vi "main OP400.vi"() -> ()   [LabVIEW 2020]
uses:
  SubVI/OP400ZP_state.ctl
  <userlib>/Alex.vi/FGV.ctl
  <vilib>/QMT/GDataBase for MySQL(tm)/MySQL/public/controls/DateType.ctl
  OP500/VG/VG_progressBar.vi
  OP600/SubVI/CheminDeBase.vi
  <vilib>/Utility/error.llb/Error Cluster From Error Code.vi
  VG/PN.vi
  VG/ZENTYPE.vi
  VG/IS30%.vi
  OP300/EN PRODUCTION/OP300-CONTI-AUTO/VG/R.vi
  VG/VG_BT3562.vi
  SubVI/OP400ZP_OCVmin.vi
  SubVI/OP400ZP_OCVmax.vi
  VG/VG_MX5060.vi
  <vilib>/Instr/_visa.llb/VISA Configure Serial Port (Instr).vi
  VG/VG_ARDUINO.vi
  <vilib>/QMT/GDataBase for MySQL(tm)/MySQL/MySQLConnector.lvclass
panel:
  out "error out":errorcluster
  out "INSERT INTO":string
  out "Revision":i32=288
  out "BDD 2":T1
  in  "arrêt":bool
  out "BT3562A":refnum<visa-resource-name>
  out "MX5060":refnum<visa-resource-name>
  in  "VISA OUT":T2
  out "VISA OUT":T2
  out "Compt":i32
  in  "DERNIER2":bool
  out "30% ?":bool
  out "SN":string
  out "Zentype":string
  out "BDD":T3
  out "Numérique":i32
  out "progression":dbl(slide) scale=0.0..1000.0
  out "PN":string
  out "errout 2":errorcluster={"status"=TRUE, "code"=0, "source"="PCAN_CHANNEL ILLEGAL"} caption="errout"
  out "errout":errorcluster caption="sortie d'erreur"
  out "STOP":bool
  out "TOP":string
  out "DRAW":picture
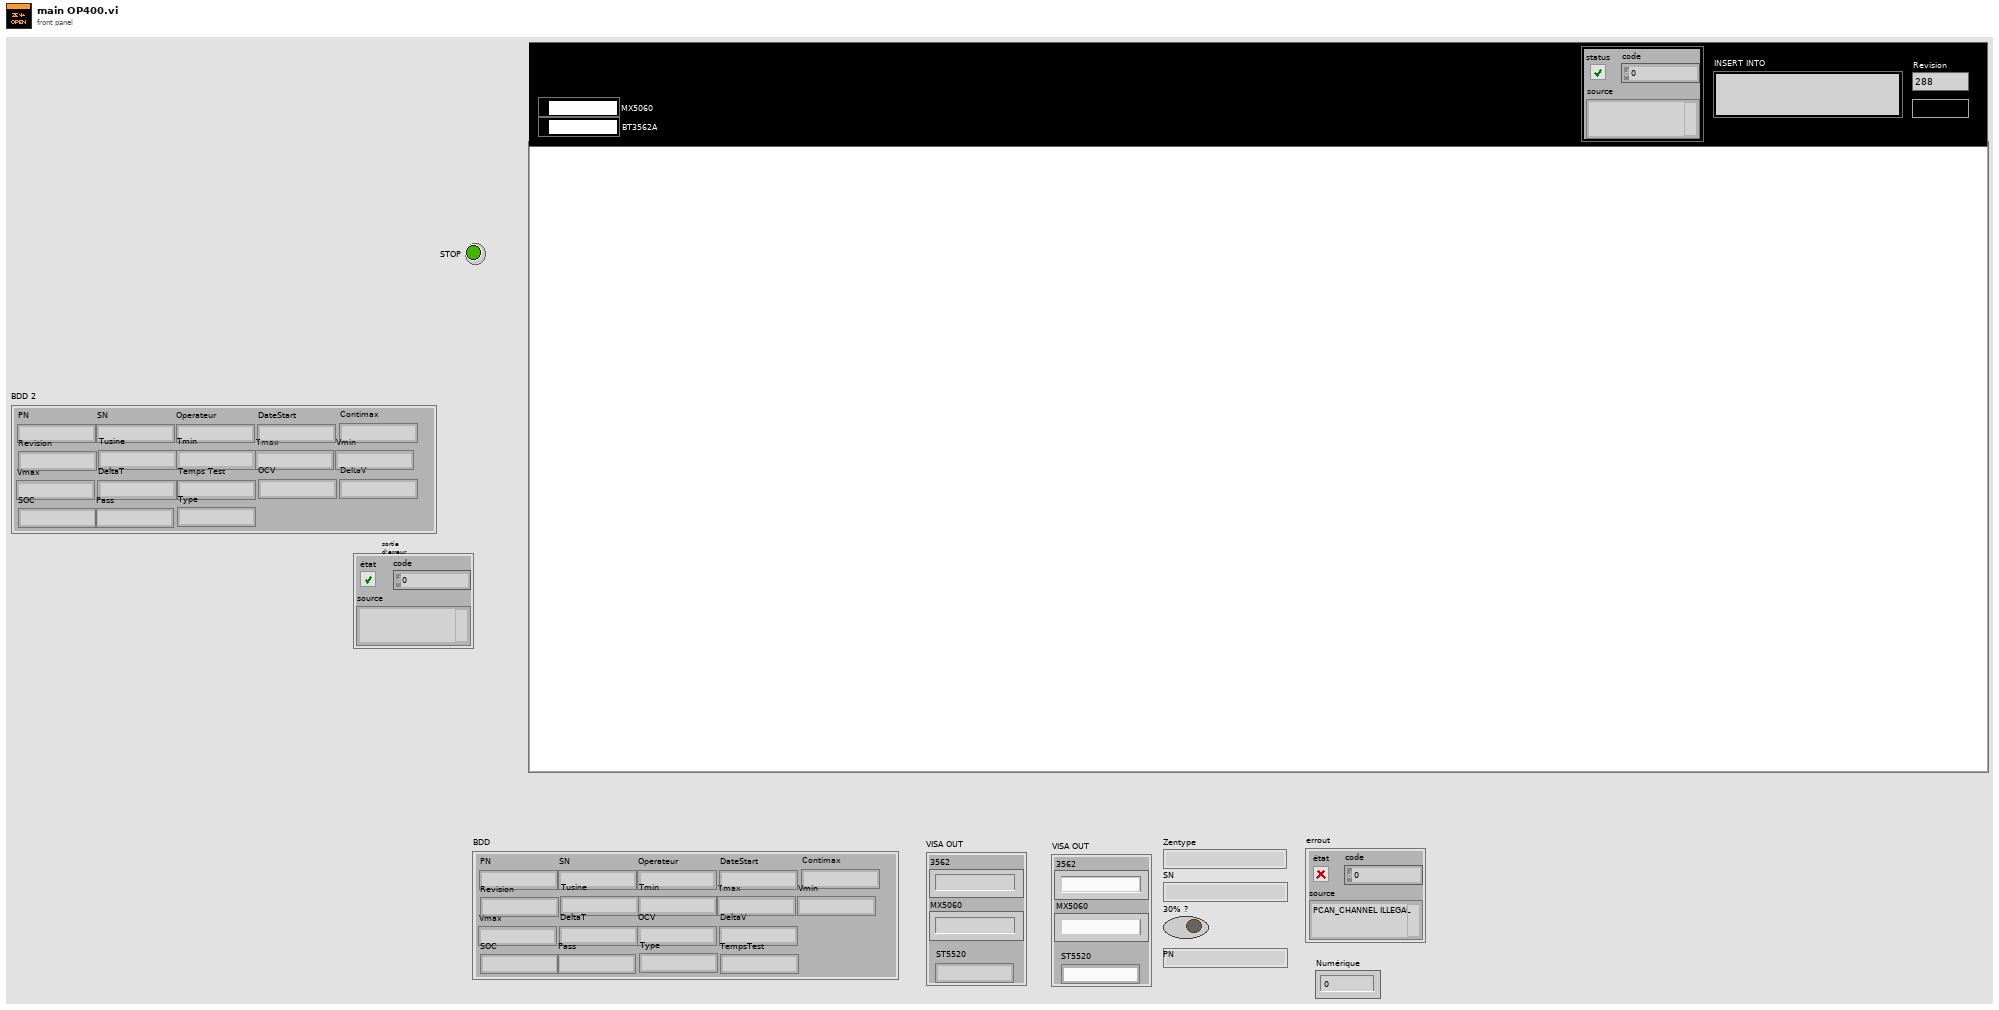
[diagram p1: front panel]
types:
  T1 = cluster{"Operateur":string, "DateStart":string, "Contimax":string, "PN":string, "Revision":string, "Tusine":string, "Tmin":string, "Tmax":string, "Vmin":string, "Vmax":string, "DeltaT":string, "Temps Test":string, "OCV":string, "SN":string, "DeltaV":string, "SOC":string, "Pass":string, "Type":string}
  T2 = cluster{"3562":string, "MX5060":string, "ST5520":string}
  T3 = cluster{"PN":string, "SN":string, "Operateur":string, "DateStart":string, "Contimax":string, "Revision":string, "Tusine":string, "Tmin":string, "Tmax":string, "Vmin":string, "Vmax":string, "DeltaT":string, "OCV":string, "DeltaV":string, "SOC":string, "Pass":string, "Type":string, "TempsTest":string}
  T4 = cluster{"PN":string, "Opérateur":string, "Sealing":string, "Conti":string, "OCV":string, "1_TCellmin":string, "1_TCellmax":string, "1_VCellmin":string, "1_VCellmax":string, "1_Nbmodule":string, "Résultat final":string, "Résultat final 2":string, "1_Nbmodule 2":string, "1_VCellmax 2":string, "Résultat final 3":string, "1_Nbmodule 3":string, "Résultat final 4":string, "1_Nbmodule 4":string, "1_VCellmax 3":string, "Résultat final 5":string}
  T5 = typedef "OP400ZP_state.ctl" = enum16{"Null", "Demarrage", "Init", "Scan", "Montage", "Conti", "Iso", "Vpack", "DataDyn", "Demontage", "Crash", "Next", "Sealing", "Comext"}
  T6 = typedef "FGV.ctl" = enum16{"GET", "SET", "RAZ"}
  T7 = typedef "MySQLVIEW.lvlib/MySQLConnector.lvclass/DateType.ctl" = enum16{"DATETIME", "DATE", "TIMESTAMP", "TIME", "YEAR (2 digits)", "YEAR (4 digits)"}
  T8 = enum32{"BT3561A", "BT3562A", "BT3563A", "BT3562", "BT3563", "BT3564", "3561"}
  T9 = cluster{"1_TCellmin":string, "1_TCellmax":string, "1_VCellmin":string, "1_VCellmax":string, "1_Nbmodule":string, "1_TUsine":string, "1_DeltaT":string, "1_DeltaV":string}
  T10 = typedef "imagedata.ctl" = cluster{"image type":i32, "image depth":i32, "image":u8[], "mask":u8[], "colors":u32[], "Rectangle":cluster{"left":i16, "top":i16, "right":i16, "bottom":i16}}
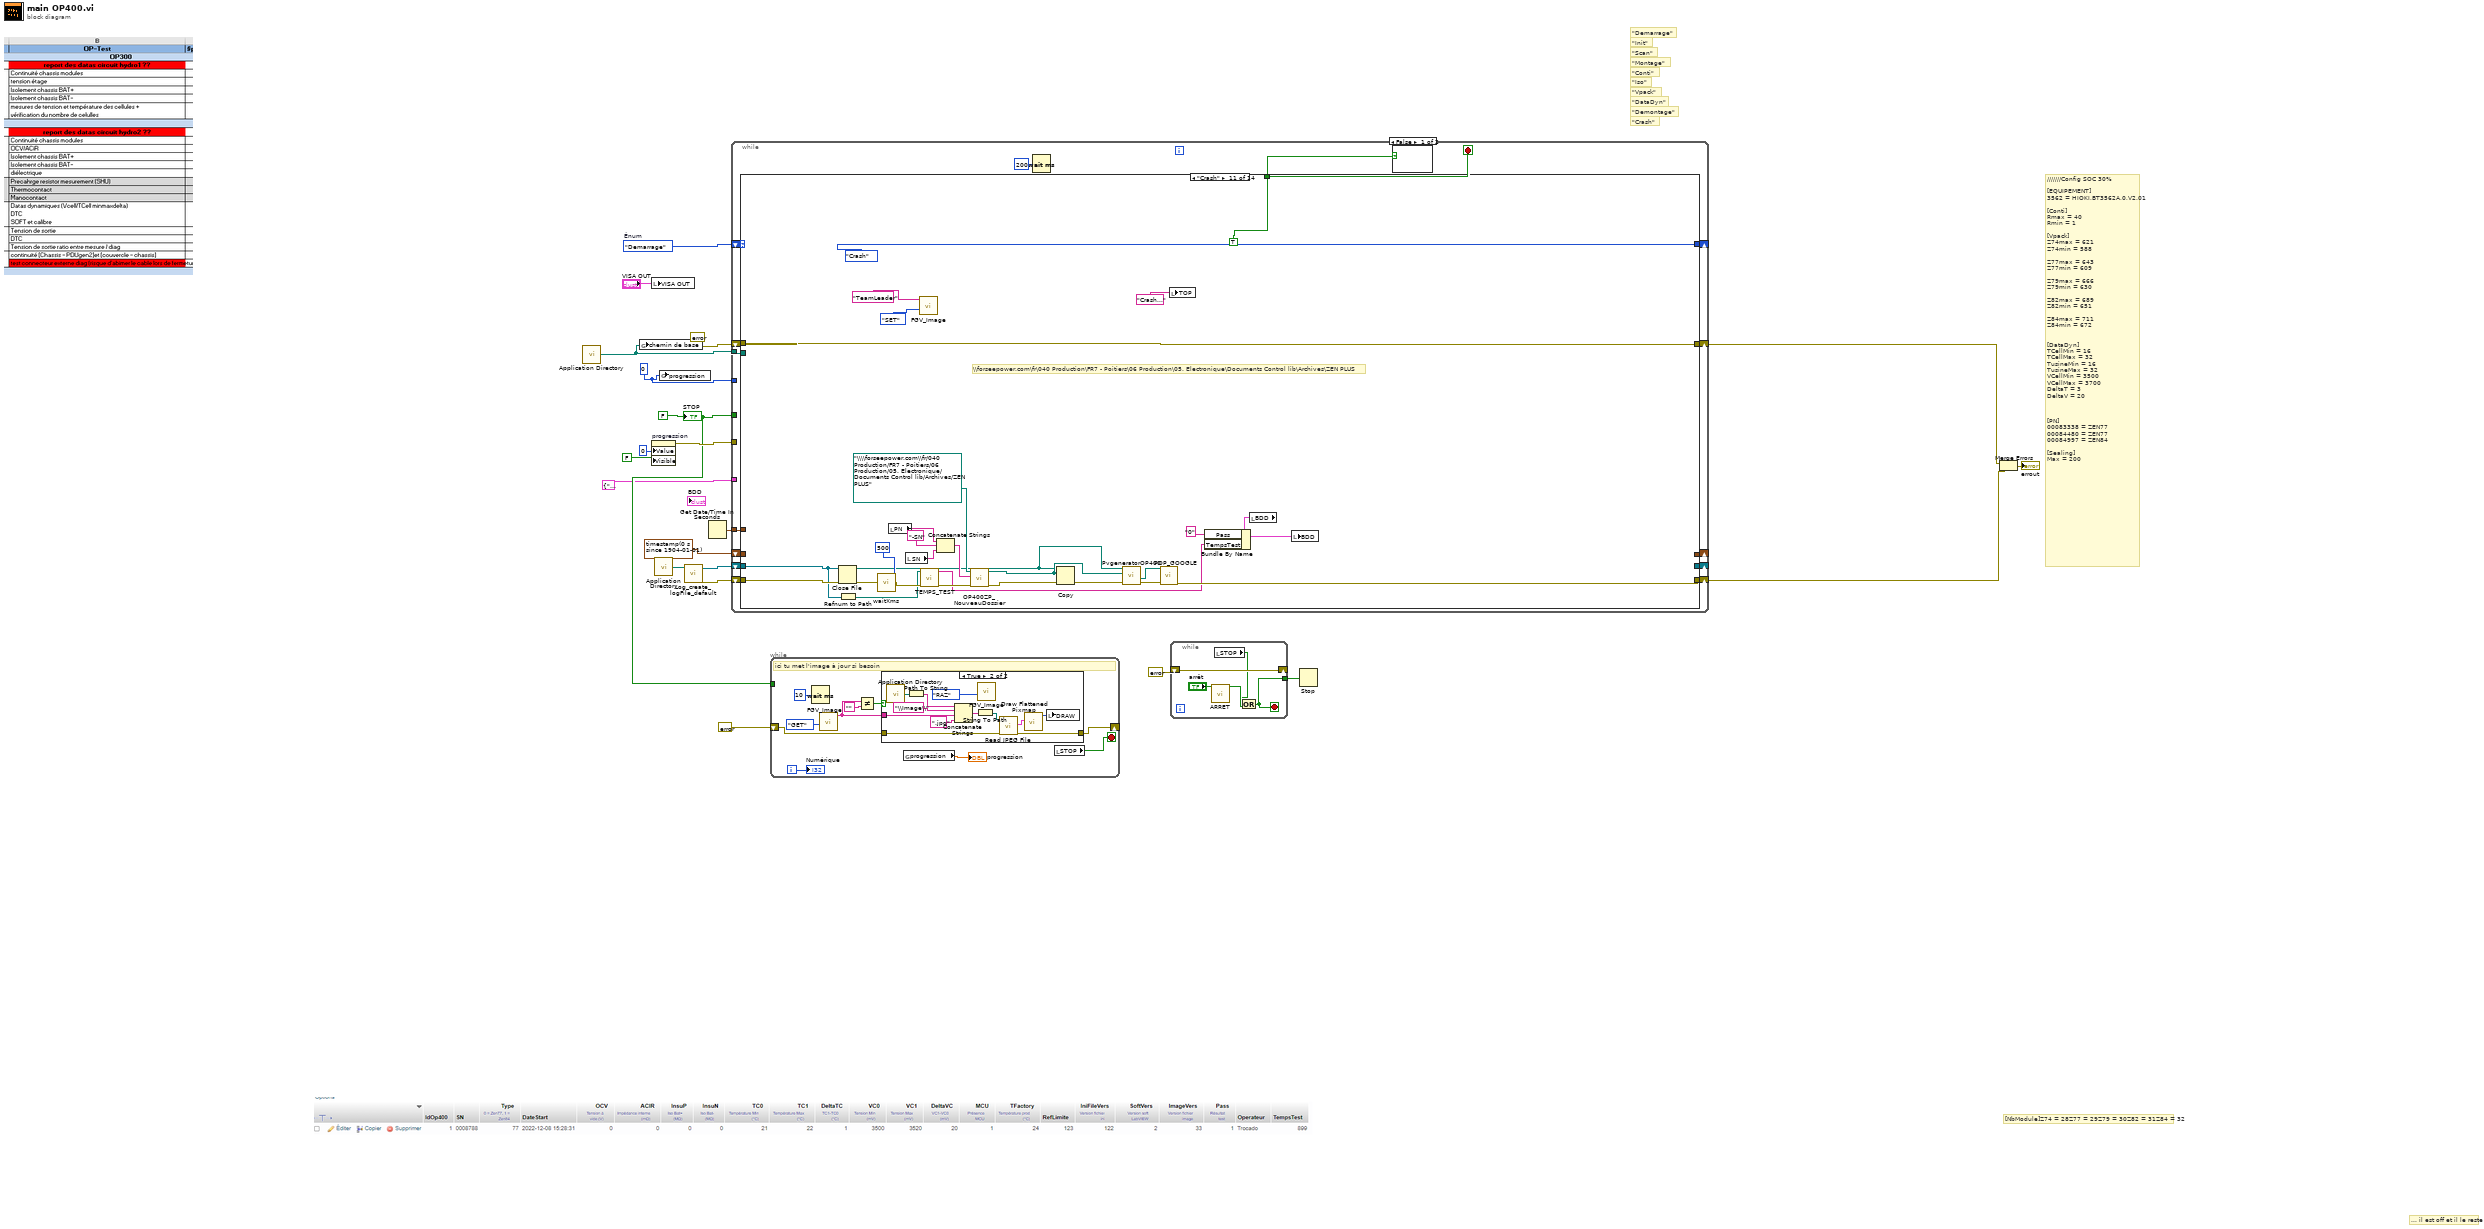
[diagram p0: block diagram]
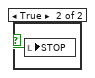
[diagram p3: hidden frame]
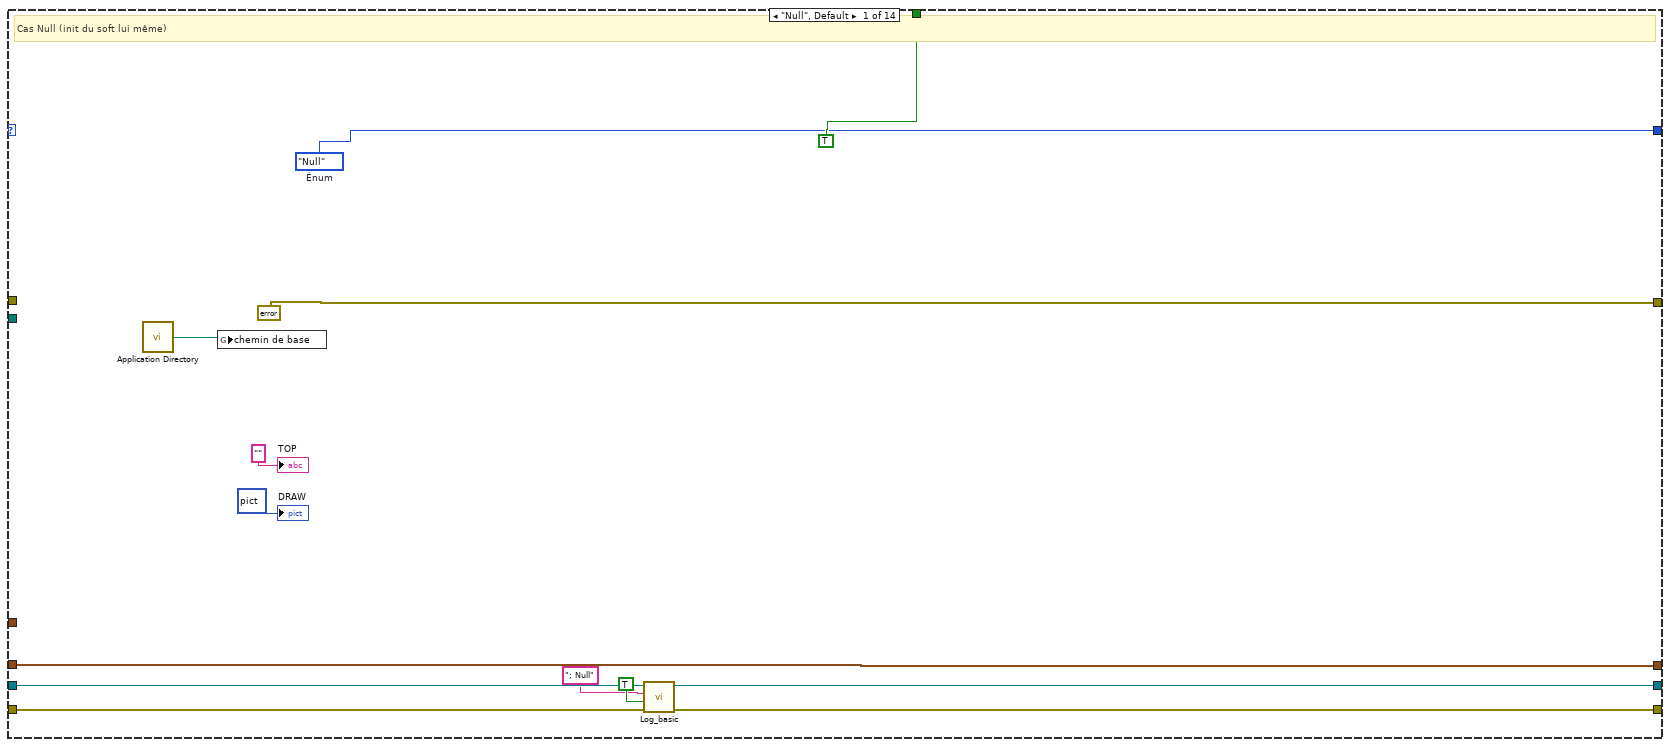
[diagram p4: hidden frame]
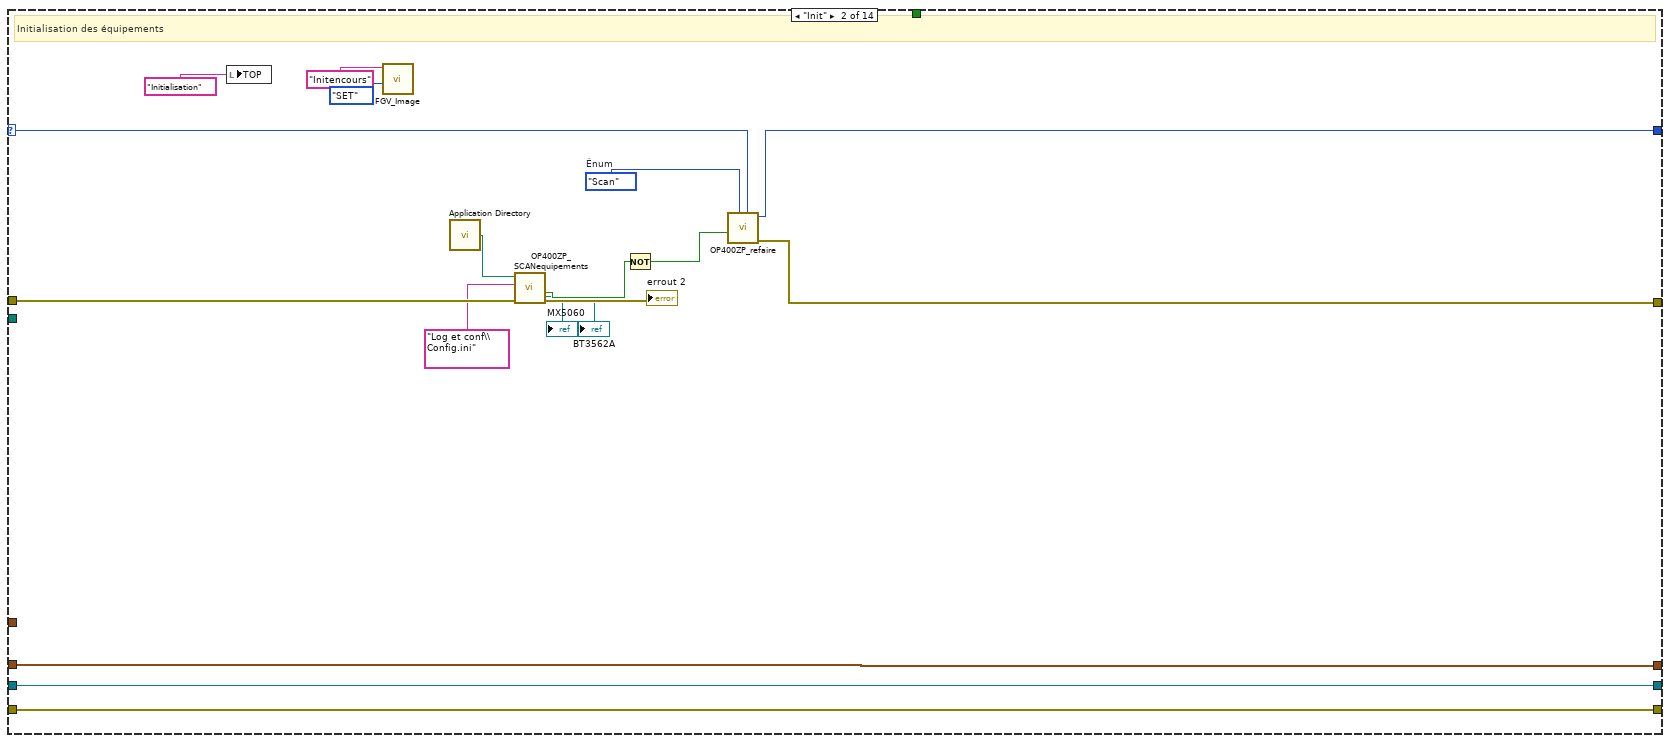
[diagram p5: hidden frame]
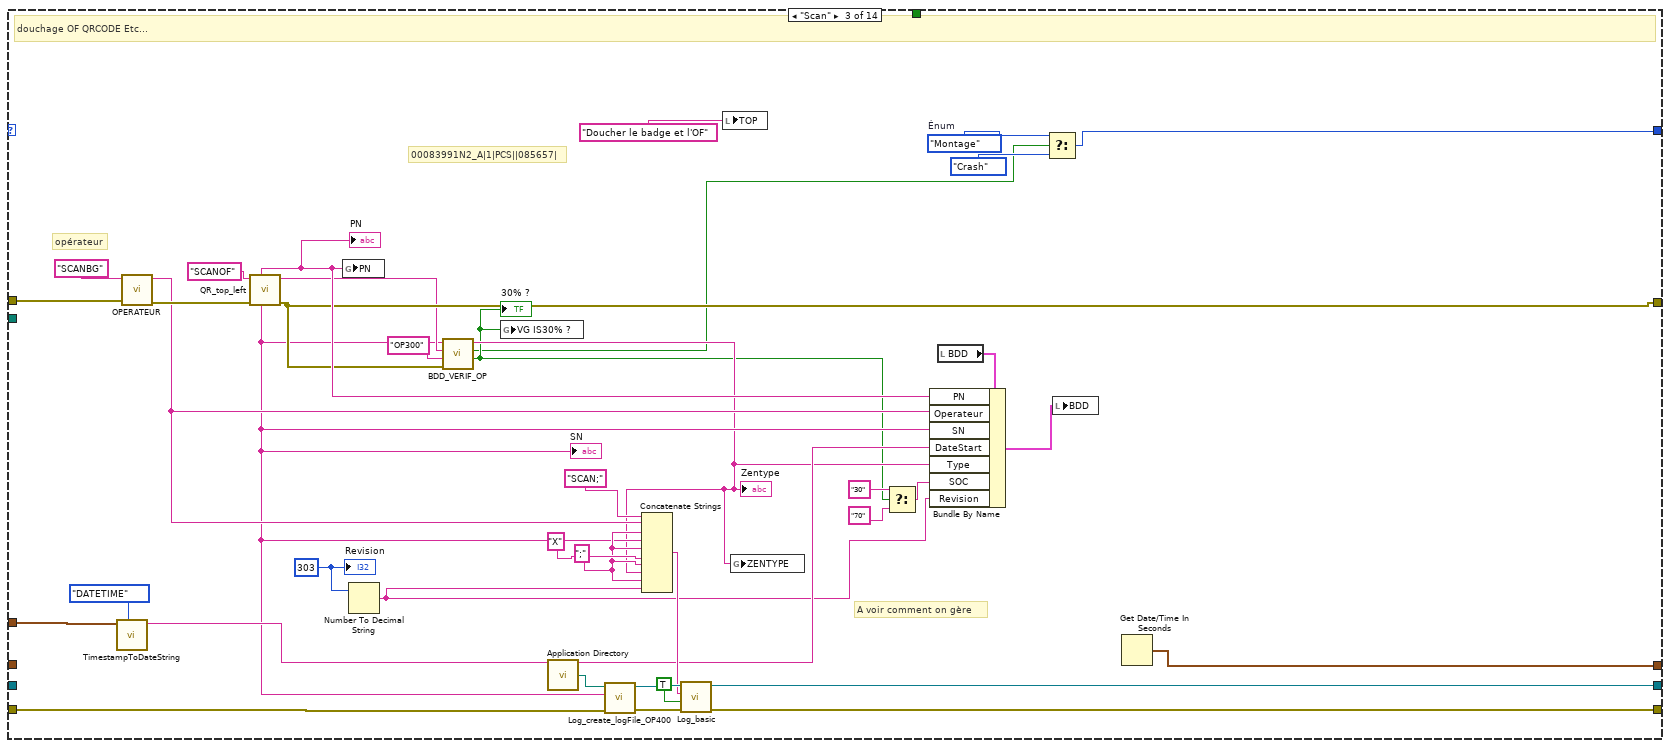
[diagram p6: hidden frame]
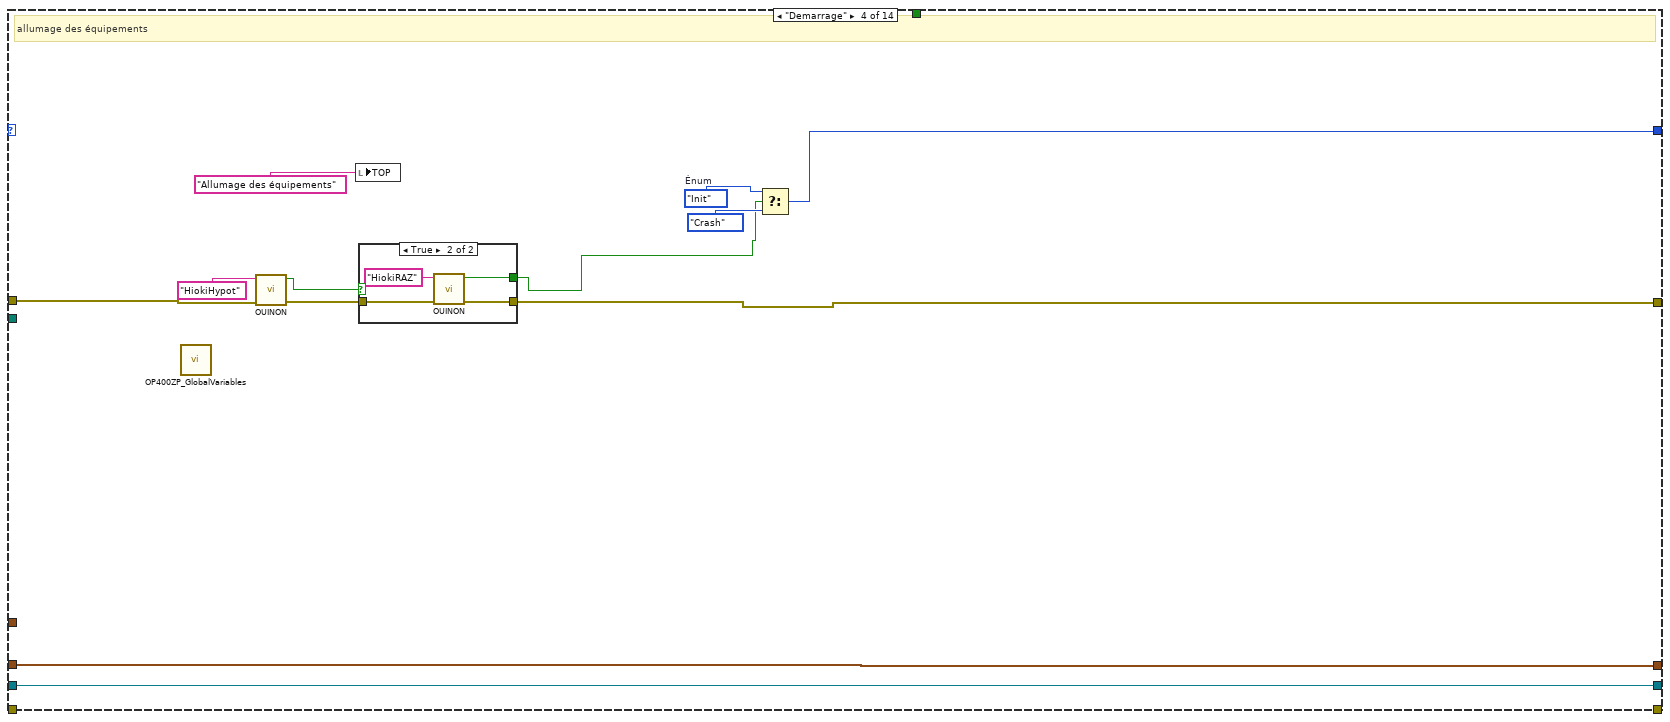
[diagram p7: hidden frame]
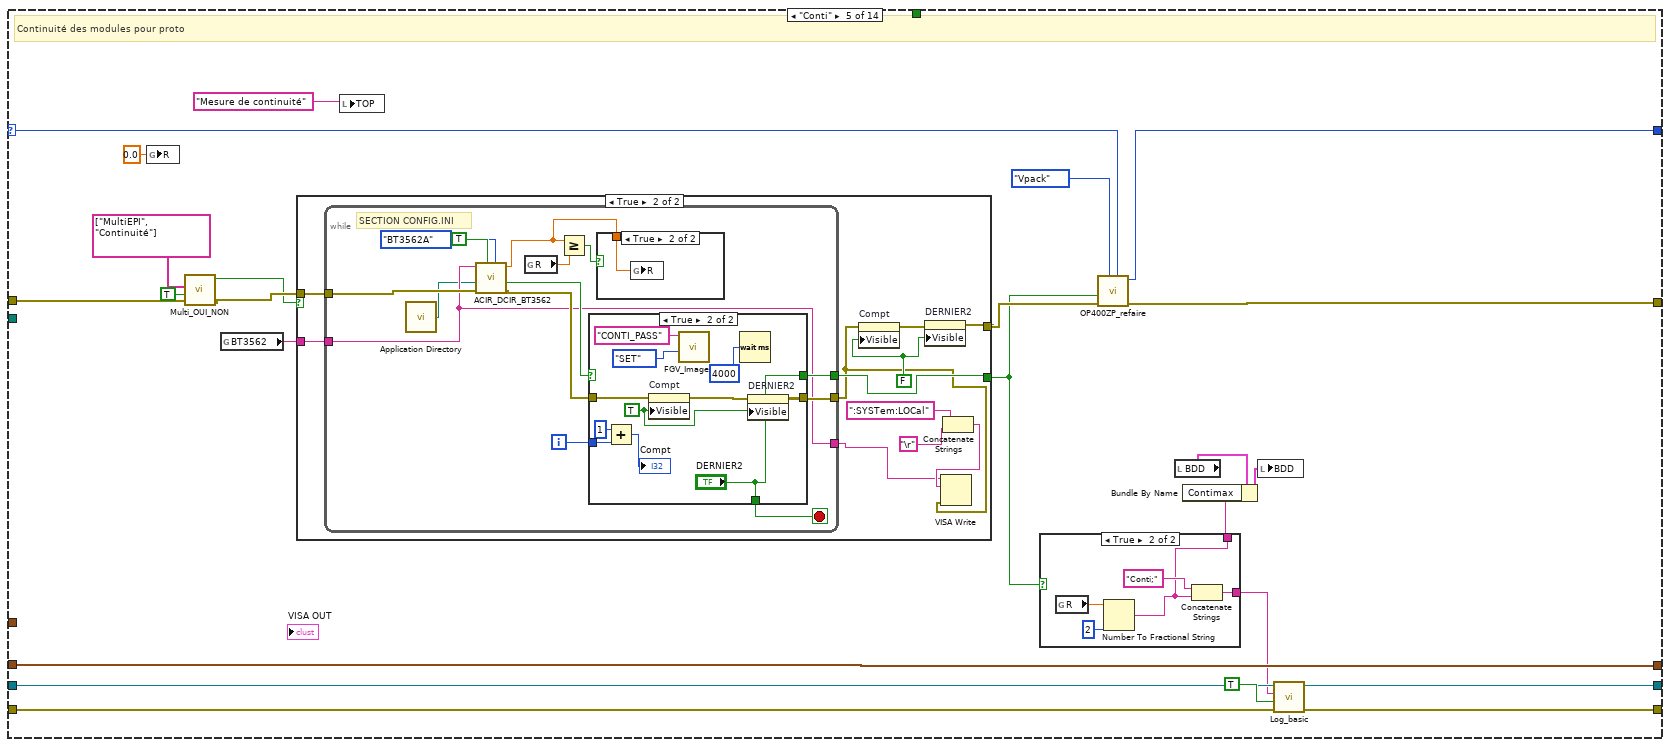
[diagram p9: hidden frame]
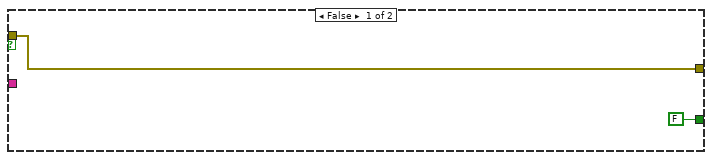
[diagram p10: hidden frame]
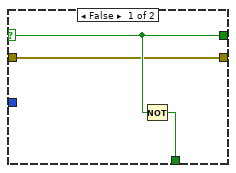
[diagram p11: hidden frame]
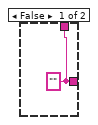
[diagram p13: hidden frame]
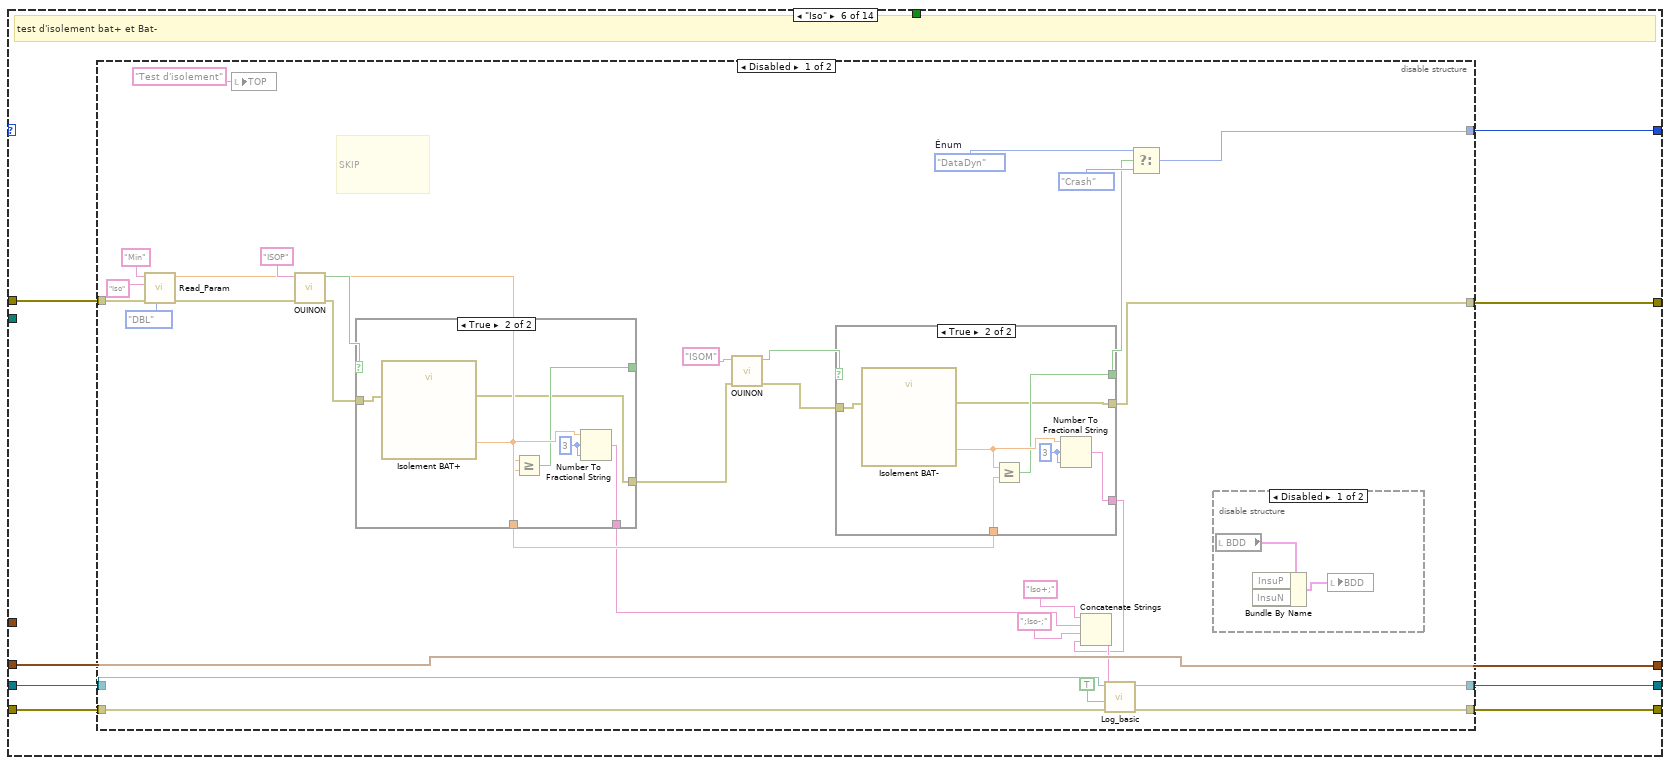
[diagram p14: hidden frame]
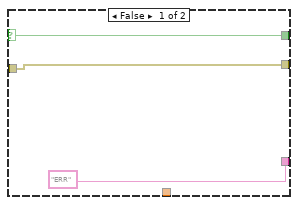
[diagram p16: hidden frame]
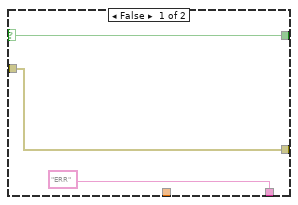
[diagram p17: hidden frame]
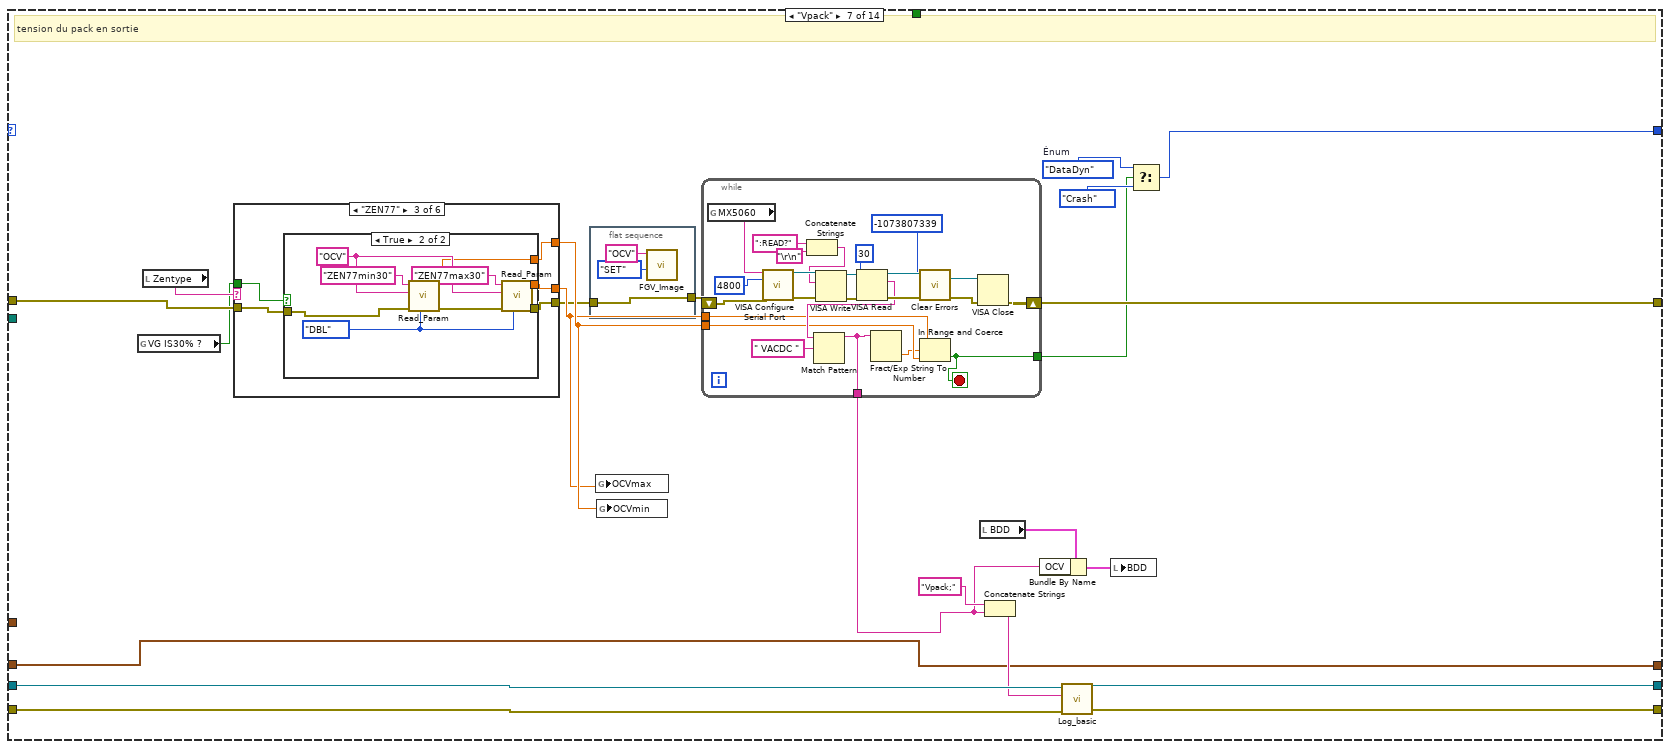
[diagram p19: hidden frame]
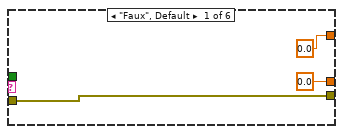
[diagram p20: hidden frame]
diagram:
  w1 = u8 0 ("progression")
  w12 = OP400ZP_state."Demarrage"  # Énum
  w7 = FALSE ("STOP")
  # "[NbModule]Z74 = 28Z77 = 29Z79 = 30Z82 = 31Z84 = 32"
  # "///////Config SOC 30%\n\n[EQUIPEMENT]\n3562 = HIOKI,BT3562A,0,V2.01\n\n[Conti]\nRmax = 40\nRmin = 1\n\n[Vpack]\nZ74max = 621\nZ74min = 588\n\nZ77max = 643\nZ77min = 609\n\nZ79max = 666\nZ79min = 630\n\nZ82max = 689\nZ82min = 651\n\nZ84max = 711\nZ84min = 672\n\n\n[DataDyn]\nTCellMin = 16\nTCellMax = 32\nTusineMin = 16\nTusineMax = 32\nVCellMin = 3500\nVCellMax = 3700\nDeltaT = 3\nDeltaV = 20\n\n\n\n[PN]\n00083338 = ZEN77\n00084480 = ZEN77\n00084997 = ZEN84\n\n[Sealing]\nMax = 200"
  # "\"Crash\""
  # "\"Demontage\""
  # "\"DataDyn\""
  # "\"Iso\""
  # "\"Montage\""
  # "\"Scan\""
  # "\"Init\""
  # "\"Demarrage\""
  # "\"Conti\""
  # "\"Vpack\""
  # "... il est off et il le reste"
  n1 = call <vilib>:"Application Directory.vi"() -> ("Application Directory"=w17:path)
  n2 = global write "CheminDeBase.vi" "chemin de base"(w17) -> ()
  n3 = local write "VISA OUT"("VISA OUT") -> ()
  n4 = property on="progression" class="Slide (strict)"("Value"=u8 0 ("progression"), "Visible"=FALSE) -> (error out=w10:errorcluster)  [unwired: 2 in, 1 out]
  n5 = call <vilib>:"Application Directory.vi"() -> ("Application Directory"=w15:path)
  n6 = global write "VG_progressBar.vi" "progression"(w1) -> ()
  n7 = call "Log_create_logFile_default.vi"("appdir"=w15) -> ("errout"=w16:errorcluster, "Fichier à flux d'octets en sortie"=w18:refnum<file>)  [unwired: 9 in]
  n8 = Get Date/Time In Seconds() -> (seconds since 1Jan1904=w2:timestamp)
  n9 = while {
    shift-right: [w34] -> w20
    shift-left: errorcluster {"status"=FALSE, "code"=0, "source"=""} ("error out") -> [w23]
    shift-right: [w27] -> _
    shift-left: w12 -> [w28]
    shift-right: [w30] -> w19
    shift-left: w16 -> [w33]
    shift-right: [w31] -> _
    shift-left: w18 -> [w32]
    tunnel: w17 -> [w26]
    tunnel: w7 -> [_]
    shift-right: [w24] -> _
    shift-left: timestamp(0 s since 1904-01-01) ("seconds since 1Jan1904") -> [w25]
    tunnel: w1 -> [_]
    tunnel: w10 -> [_]
    tunnel: T4 {"PN"="", "Opérateur"="", "Sealing"="", "Conti"="", "OCV"="", "1_TCellmin"="", "1_TCellmax"="", "1_VCellmin"="", "1_VCellmax"="", "1_Nbmodule"="", "Résultat final"="", "Résultat final 2"="", "1_Nbmodule 2"="", "1_VCellmax 2"="", "Résultat final 3"="", "1_Nbmodule 3"="", "Résultat final 4"="", "1_Nbmodule 4"="", "1_VCellmax 3"="", "Résultat final 5"=""} ("Cluster") -> [_]
    tunnel: w2 -> [w22]
    stop <- w29 stop-if-true
    n10 = case shown="\"Crash\"" w28 {
      selector: w28 -> [_ w62 _ _ w140 _ _ w461 _ _ _ _ _ w669]
      tunnel: w23 -> [_ w64 w84 w117 w129 w204 w268 w433 w537 w556 w585 w614 w616 w665]
      tunnel: [errorcluster {"status"=FALSE, "code"=0, "source"=""} ("errin") w58 w74 w108 w142 w203 w273 w437 w536 w550 w585 w613 w619 w668] -> w34
      tunnel: w33 -> [w45 w67 w103 _ w147 w201 w277 w467 w534 w543 w577 w610 w623 w674]
      tunnel: w32 -> [w46 w66 _ w118 w146 w200 w276 w468 w535 w541 w561 w611 w621 w673]
      tunnel: [w43 w66 w105 w118 w145 w199 w275 w465 w535 w541 _ _ w620 w672] -> w31
      tunnel: [w44 w67 w106 _ w144 w202 w274 w466 w534 w542 w565 w595 w622 w671] -> w30
      tunnel: [TRUE _ _ _ _ _ _ _ _ w558 TRUE _ _ _] -> w29
      tunnel: [w37 w63 w93 w110 w139 w197 w269 w460 w530 w552 OP400ZP_state."Crash" w612 w618 w670] -> w27
      tunnel: w26 -> [_ _ _ _ _ _ _ _ _ _ _ _ _ w667]
      tunnel: w25 -> [w39 w65 _ w116 w143 w198 w270 w462 w533 w555 _ _ w617 w662]
      tunnel: [w39 w65 w97 w116 w143 w198 w270 w462 w533 w555 _ _ w617 w663] -> w24
      tunnel: w22 -> [_ _ w79 _ _ _ _ _ _ _ _ _ _ _]
      frame "Null", Default {
        w37 = OP400ZP_state."Null"  # Énum
        # "Cas Null (init du soft lui même)"
        n11 = call <vilib>:"Application Directory.vi"() -> ("Application Directory"=w49:path)
        n12 = global write "CheminDeBase.vi" "chemin de base"(w49) -> ()
        n13 = call "Log_basic.vi"("errin"=w45, "date?"=TRUE, "chaîne"="; Null", "in"=w46) -> ("sortie d'erreur"=w44:errorcluster, "refnum en sortie"=w43:refnum<file>)  [unwired: 6 in]
        "DRAW" <- picture data[5B] ("DRAW")
        "TOP" <- "" ("TOP")
      }
      frame "Init" {
        w53 = OP400ZP_state."Scan"  # Énum
        # "Initialisation des équipements"
        n14 = local write "TOP"("Initialisation" ("TOP")) -> ()
        n15 = call <userlib>:"FGV_Image.vi"("Énum"=FGV."SET", "IN"="Initencours") -> ()  [unwired: 9 in, 1 out]
        n16 = call <vilib>:"Application Directory.vi"() -> ("Application Directory"=w56:path)
        n17 = call "OP400ZP_SCANequipements.vi"("Errin"=w64, "Chaîne"="Log et conf\\Config.ini", "pathin"=w56) -> ("errout"=→"errout 2":errorcluster, "KO?"=w54:bool, "BT"=→"BT3562A":refnum<visa-resource-name>, "MX"=→"MX5060":refnum<visa-resource-name>)  [unwired: 5 in]
        n18 = Not(x=w54) -> (.not. x?=w55:bool)
        n19 = call "OP400ZP_refaire.vi"("refaire"=w62, "Cas OK"=w53, "test ok ?"=w55) -> ("errout"=w58:errorcluster, "OUT"=w63:T5)  [unwired: 7 in]
      }
      frame "Scan" {
        w76 = 303
        w92 = OP400ZP_state."Montage"  # Énum
        w83 = ";" ("chaîne")
        # "A voir comment on gère"
        # "00083991N2_A|1|PCS||085657|"
        # "opérateur"
        # "douchage OF QRCODE Etc..."
        n20 = call <vilib>:"TimestampToDateString.vi"("dateType"=DateType."DATETIME", "timestamp in"=w79) -> ("dateString"=w78:string)  [unwired: 8 in, 1 out]
        n21 = call <userlib>:"OPERATEUR.vi"("errin"=w84, "IN"="SCANBG") -> ("error out"=w96:errorcluster, "Dataout"=w87:string)  [unwired: 8 in]
        n22 = call <userlib>:"QR_top_left.vi"("errin"=w96, "image"="SCANOF") -> ("error out"=w74:errorcluster, "Réponse"=w73:string, "SN"=w72:string, "PN"=w85:string)  [unwired: 5 in, 1 out]
        "PN" <- w85
        "SN" <- w72
        n23 = global write "PN.vi" "PN"(w85) -> ()
        n24 = Number To Decimal String(number=w76) -> (decimal integer string=w75:string)  [unwired: 1 in]
        n25 = call <userlib>:"BDD_VERIF_OP.vi"("errin"=w74, "N°OPVerif?"="OP300", "OF"=w73, "SN"=w72) -> ("IS30% ?"=w69:bool, "Continue?"=w68:bool, "TYPE"=w70:string)  [unwired: 4 in, 1 out]
        "Zentype" <- w70
        "30% ?" <- w69
        n26 = global write "IS30%.vi" "VG IS30% ?"(w69) -> ()
        n27 = call <vilib>:"Application Directory.vi"() -> ("Application Directory"=w104:path)
        n28 = call "Log_create_logFile_OP400.vi"("errin"=w103, "toute l'expression"=w72, "Application Directory"=w104) -> ("sortie d'erreur"=w101:errorcluster, "Fichier à flux d'octets en sortie"=w102:refnum<file>)  [unwired: 7 in]
        n29 = Concatenate Strings("SCAN;" ("chaîne"), w87, w83, w72, w83, "X" ("chaîne"), w83, w70, w83, w75) -> (w99:string)
        n30 = call "Log_basic.vi"("errin"=w101, "date?"=TRUE, "chaîne"=w99, "in"=w102) -> ("sortie d'erreur"=w106:errorcluster, "refnum en sortie"=w105:refnum<file>)  [unwired: 6 in]
        n31 = local write "TOP"("Doucher le badge et l'OF" ("TOP")) -> ()
        n32 = global write "ZENTYPE.vi" "ZENTYPE"(w70) -> ()
        n33 = Select(t="30", s=w69, f="70") -> (s? t:f=w80:string)
        n34 = local read "BDD"() -> (w88:T3)
        n35 = Bundle By Name(cluster=w88, "PN"=w85, "Operateur"=w87, "SN"=w72, "DateStart"=w78, "Type"=w70, "SOC"=w80, "Revision"=w75) -> (w89:T3)
        n36 = Select ("Sélectionner")(t=w92, s=w68, f=OP400ZP_state."Crash" ("cas faux")) -> (s? t:f=w93:T5)
        n37 = local write "BDD"(w89) -> ()
        n38 = Get Date/Time In Seconds() -> (seconds since 1Jan1904=w97:timestamp)
        "Revision" <- w76
      }
      frame "Demarrage" {
        w111 = OP400ZP_state."Init"  # Énum
        # "allumage des équipements"
        n39 = call "OP400ZP_GlobalVariables.vi"() -> ()  [unwired: 12 in]
        n40 = call "OUINON.vi"("errin"=w117, "image"="HiokiHypot") -> ("error out"=w114:errorcluster, "OUI/NON"=w113:bool)  [unwired: 8 in]
        n41 = local write "TOP"("Allumage des équipements" ("TOP")) -> ()
        n42 = case shown="True" w113 {
          selector: w113 -> [w120 _]
          tunnel: [w120 w124] -> w107
          tunnel: [w119 w123] -> w108
          tunnel: w114 -> [w119 w121]
          frame False {
          }
          frame True {
            n43 = call "OUINON.vi"("errin"=w121, "image"="HiokiRAZ" ("IN")) -> ("error out"=w123:errorcluster, "OUI/NON"=w124:bool)  [unwired: 8 in]
          }
        }
        n44 = Select ("Sélectionner")(t=w111, s=w107, f=OP400ZP_state."Crash" ("cas faux")) -> (s? t:f=w110:T5)
      }
      frame "Conti" {
        # "Continuité des modules pour proto"
        n45 = global write "R.vi" "R"(0.0 ("R")) -> ()
        n46 = call "Multi_OUI_NON.vi"("errin"=w129, "errinb"=TRUE, "Tableau"=string[] ["MultiEPI", "Continuité"]) -> ("errout"=w128:errorcluster, "isok?"=w127:bool)  [unwired: 7 in]
        n47 = global read "VG_BT3562.vi" "BT3562"() -> (w131:string)
        n48 = case shown="True" w127 {
          tunnel: w128 -> [w150 w161]
          tunnel: [w150 w159] -> w132
          tunnel: [FALSE ("OUI/NON") w160] -> w125
          tunnel: w131 -> [_ w156]
          frame False {
          }
          frame True {
            w157 = FALSE ("Visible")
            n49 = while {
              tunnel: w156 -> [w165]
              tunnel: w161 -> [w175]
              tunnel: [w173] -> w151
              tunnel: [w168] -> w160
              tunnel: [w165] -> w152
              i -> [w172]
              stop <- w167 stop-if-true
              # "SECTION CONFIG.INI"
              n50 = call <vilib>:"Application Directory.vi"() -> ("Application Directory"=w164:path)
              n51 = call <userlib>:"ACIR_DCIR_BT3562.vi"("Model"=T8."BT3562A", "juste R?"=TRUE, "errin"=w175, "chemin de base"=w164, "VISAin"=w165) -> ("errout"=w166:errorcluster, "OK?"=w174:bool, "R"=w169:dbl)  [unwired: 1 in, 3 out]
              n52 = global read "R.vi" "R"() -> (w171:dbl)
              n53 = Greater Or Equal?(x=w169, y=w171) -> (x >= y?=w170:bool)
              n54 = case shown="True" w174 {
                selector: w174 -> [w178 _]
                tunnel: w166 -> [w176 w185]
                tunnel: [w176 w181] -> w173
                tunnel: [w177 "DERNIER2"] -> w167
                tunnel: w172 -> [_ w187]
                tunnel: [w178 "DERNIER2"] -> w168
                frame False {
                  n55 = Not(x=w178) -> (.not. x?=w177:bool)
                }
                frame True {
                  w179 = TRUE ("Visible")
                  n56 = Add(x=1, y=w187) -> (x+y=→"Compt":i32)
                  n57 = property on="Compt" class="DigNum (strict)"(error in=w185, "Visible"=w179) -> (error out=w182:errorcluster)  [unwired: 1 in, 1 out]
                  n58 = call <userlib>:"FGV_Image.vi"("Énum"=FGV."SET", "IN"="CONTI_PASS") -> ()  [unwired: 9 in, 1 out]
                  n59 = Wait (ms)(milliseconds to wait=u32 4000 ("attente (ms)")) -> ()  [unwired: 1 out]
                  n60 = property on="DERNIER2" class="Bool"(error in=w182, "Visible"=w179) -> (error out=w181:errorcluster)  [unwired: 1 in, 1 out]
                }
              }
              n61 = case shown="True" w170 {
                tunnel: w169 -> [_ w190]
                frame False {
                }
                frame True {
                  n62 = global write "R.vi" "R"(w190) -> ()
                }
              }
            }
            n63 = property on="Compt" class="DigNum (strict)"(error in=w151, "Visible"=w157) -> (error out=w158:errorcluster)  [unwired: 1 in, 1 out]
            n64 = property on="DERNIER2" class="Bool"(error in=w158, "Visible"=w157) -> (error out=w159:errorcluster)  [unwired: 1 in, 1 out]
            n65 = Concatenate Strings(":SYSTem:LOCal" ("write buffer"), "\r") -> (w154:string)
            n66 = VISA Write(VISA resource name=w152, write buffer=w154, error in (no error)=w151) -> ()  [unwired: 3 out]
          }
        }
        n67 = local write "TOP"("Mesure de continuité" ("TOP")) -> ()
        n68 = case shown="True" w125 {
          tunnel: [w191 w193] -> w133
          tunnel: [w191 w192] -> w134
          frame False {
            w191 = ""
          }
          frame True {
            n69 = global read "R.vi" "R"() -> (w195:dbl)
            n70 = Number To Fractional String(number=w195, precision (6)=i16 2 ("précision (6)")) -> (F-format string=w192:string)  [unwired: 2 in]
            n71 = Concatenate Strings("Conti;" ("chaîne"), w192) -> (w193:string)
          }
        }
        n72 = call "OP400ZP_refaire.vi"("refaire"=w140, "Cas OK"=OP400ZP_state."Vpack" ("Énum"), "errin"=w132, "test ok ?"=w125) -> ("errout"=w142:errorcluster, "OUT"=w139:T5)  [unwired: 6 in]
        n73 = local read "BDD"() -> (w136:T3)
        n74 = Bundle By Name(cluster=w136, "Contimax"=w134) -> (w135:T3)
        n75 = local write "BDD"(w135) -> ()
        n76 = call "Log_basic.vi"("errin"=w147, "date?"=TRUE, "chaîne"=w133, "in"=w146) -> ("sortie d'erreur"=w144:errorcluster, "refnum en sortie"=w145:refnum<file>)  [unwired: 6 in]
      }
      frame "Iso" {
        # "test d'isolement bat+ et Bat-"
        n77 = disable-structure shown="Disabled" {
          disable-tunnel: w204 -> [w226 _]
          disable-tunnel: [w221 _] -> w203
          disable-tunnel: [w217 _] -> w202
          disable-tunnel: w201 -> [w216 _]
          disable-tunnel: w200 -> [w215 _]
          disable-tunnel: [w214 _] -> w199
          disable-tunnel: [w209 _] -> w197
          frame Disabled {
            w211 = OP400ZP_state."DataDyn"  # Énum
            # "SKIP"
            n78 = call <userlib>:"Read_Param.vi"("Énum"=enum16{"STR", "DBL", "U32"}."DBL", "errin"=w226, "section"="Iso", "key"="Min") -> ("error out"=w225:errorcluster, "dbl"=w219:dbl)  [unwired: 3 in, 3 out]
            n79 = local write "TOP"("Test d'isolement" ("TOP")) -> ()
            n80 = call "OUINON.vi"("errin"=w225, "image"="ISOP" ("IN")) -> ("error out"=w231:errorcluster, "OUI/NON"=w232:bool)  [unwired: 8 in]
            n81 = case shown="True" w232 {
              selector: w232 -> [w246 _]
              tunnel: w231 -> [w248 w255]
              tunnel: [w248 w249] -> w223
              tunnel: ["ERR" w253] -> w206
              tunnel: [w246 w250] -> _
              tunnel: w219 -> [_ w252]
              frame False {
              }
              frame True {
                w254 = i16 3 ("largeur (-)")
                n82 = call "Isolement BAT+"("error in (no error)"=w255) -> ("ISOP"=w251:dbl, "error out"=w249:errorcluster)  [unwired: 16 in, 1 out]
                n83 = Greater Or Equal?(x=w251, y=w252) -> (x >= y?=w250:bool)
                n84 = Number To Fractional String(number=w251, width (-)=w254, precision (6)=w254) -> (F-format string=w253:string)  [unwired: 1 in]
              }
            }
            n85 = call "OUINON.vi"("errin"=w223, "image"="ISOM" ("IN")) -> ("error out"=w222:errorcluster, "OUI/NON"=w220:bool)  [unwired: 8 in]
            n86 = case shown="True" w220 {
              selector: w220 -> [w236 _]
              tunnel: w222 -> [w238 w245]
              tunnel: [w238 w239] -> w221
              tunnel: ["ERR" w243] -> w205
              tunnel: [w236 w240] -> w210
              tunnel: w219 -> [_ w242]
              frame False {
              }
              frame True {
                w244 = i16 3 ("largeur (-)")
                n87 = call "Isolement BAT-"("error in (no error)"=w245) -> ("ISOM"=w241:dbl, "error out"=w239:errorcluster)  [unwired: 16 in, 1 out]
                n88 = Greater Or Equal?(x=w241, y=w242) -> (x >= y?=w240:bool)
                n89 = Number To Fractional String(number=w241, width (-)=w244, precision (6)=w244) -> (F-format string=w243:string)  [unwired: 1 in]
              }
            }
            n90 = Concatenate Strings("Iso+;" ("chaîne"), w206, ";Iso-;" ("chaîne"), w205) -> (w230:string)
            n91 = call "Log_basic.vi"("errin"=w216, "date?"=TRUE, "chaîne"=w230, "in"=w215) -> ("sortie d'erreur"=w217:errorcluster, "refnum en sortie"=w214:refnum<file>)  [unwired: 6 in]
            n92 = Select ("Sélectionner")(t=w211, s=w210, f=OP400ZP_state."Crash" ("cas faux")) -> (s? t:f=w209:T5)
            n93 = disable-structure shown="Disabled" {
              frame Disabled {
                n94 = local read "BDD"() -> (w235:T3)
                n95 = Bundle By Name(cluster=w235) -> (w234:T3)  [unwired: 2 in]
                n96 = local write "BDD"(w234) -> ()
              }
              frame Enabled {
              }
            }
          }
          frame Enabled {
          }
        }
      }
      frame "Vpack" {
        w264 = OP400ZP_state."DataDyn"  # Énum
        # "tension du pack en sortie"
        n97 = global read "IS30%.vi" "VG IS30% ?"() -> (w259:bool)
        n98 = local read "Zentype"() -> (w260:string)
        n99 = case shown="\"ZEN77\"" w260 {
          tunnel: w268 -> [w306 w311 w334 w357 w380 w403]
          tunnel: [w306 w310 w331 w354 w379 w402] -> w258
          tunnel: [0.0 ("dbl") w309 w332 w355 w378 w401] -> w261
          tunnel: [0.0 ("dbl") w308 w333 w356 w377 w400] -> w262
          tunnel: w259 -> [_ w307 w330 w353 w376 w399]
          frame "Faux", Default {
          }
          frame "ZEN74" {
            n100 = case shown="True" w307 {
              tunnel: w311 -> [w315 w327]
              tunnel: [w313 w326] -> w310
              tunnel: [w314 w322] -> w309
              tunnel: [w312 w321] -> w308
              frame False {
                w316 = enum16{"STR", "DBL", "U32"}."DBL" ("Énum")
                w318 = "OCV" ("section")
                n101 = call <userlib>:"Read_Param.vi"("Énum"=w316, "errin"=w315, "section"=w318, "key"="ZEN74min70") -> ("error out"=w319:errorcluster, "dbl"=w312:dbl)  [unwired: 3 in, 3 out]
                n102 = call <userlib>:"Read_Param.vi"("Énum"=w316, "errin"=w319, "section"=w318, "key"="ZEN74max70") -> ("error out"=w313:errorcluster, "dbl"=w314:dbl)  [unwired: 3 in, 3 out]
              }
              frame True {
                w323 = enum16{"STR", "DBL", "U32"}."DBL" ("Énum")
                w325 = "OCV" ("section")
                n103 = call <userlib>:"Read_Param.vi"("Énum"=w323, "errin"=w327, "section"=w325, "key"="ZEN74min30") -> ("error out"=w328:errorcluster, "dbl"=w321:dbl)  [unwired: 3 in, 3 out]
                n104 = call <userlib>:"Read_Param.vi"("Énum"=w323, "errin"=w328, "section"=w325, "key"="ZEN74max30") -> ("error out"=w326:errorcluster, "dbl"=w322:dbl)  [unwired: 3 in, 3 out]
              }
            }
          }
          frame "ZEN77" {
            n105 = case shown="True" w330 {
              tunnel: w334 -> [w338 w347]
              tunnel: [w337 w346] -> w333
              tunnel: [w336 w345] -> w332
              tunnel: [w335 w344] -> w331
              frame False {
                w339 = enum16{"STR", "DBL", "U32"}."DBL" ("Énum")
                w341 = "OCV" ("section")
                n106 = call <userlib>:"Read_Param.vi"("Énum"=w339, "errin"=w338, "section"=w341, "key"="ZEN77min70") -> ("error out"=w342:errorcluster, "dbl"=w337:dbl)  [unwired: 3 in, 3 out]
                n107 = call <userlib>:"Read_Param.vi"("Énum"=w339, "errin"=w342, "section"=w341, "key"="ZEN77max70") -> ("error out"=w335:errorcluster, "dbl"=w336:dbl)  [unwired: 3 in, 3 out]
              }
              frame True {
                w348 = enum16{"STR", "DBL", "U32"}."DBL" ("Énum")
                w350 = "OCV" ("section")
                n108 = call <userlib>:"Read_Param.vi"("Énum"=w348, "errin"=w347, "section"=w350, "key"="ZEN77min30") -> ("error out"=w351:errorcluster, "dbl"=w346:dbl)  [unwired: 3 in, 3 out]
                n109 = call <userlib>:"Read_Param.vi"("Énum"=w348, "errin"=w351, "section"=w350, "key"="ZEN77max30") -> ("error out"=w344:errorcluster, "dbl"=w345:dbl)  [unwired: 3 in, 3 out]
              }
            }
          }
          frame "ZEN79" {
            n110 = case shown="True" w353 {
              tunnel: w357 -> [w361 w370]
              tunnel: [w360 w369] -> w356
              tunnel: [w359 w368] -> w355
              tunnel: [w358 w367] -> w354
              frame False {
                w362 = enum16{"STR", "DBL", "U32"}."DBL" ("Énum")
                w364 = "OCV" ("section")
                n111 = call <userlib>:"Read_Param.vi"("Énum"=w362, "errin"=w361, "section"=w364, "key"="ZEN79min70") -> ("error out"=w365:errorcluster, "dbl"=w360:dbl)  [unwired: 3 in, 3 out]
                n112 = call <userlib>:"Read_Param.vi"("Énum"=w362, "errin"=w365, "section"=w364, "key"="ZEN79max70") -> ("error out"=w358:errorcluster, "dbl"=w359:dbl)  [unwired: 3 in, 3 out]
              }
              frame True {
                w371 = enum16{"STR", "DBL", "U32"}."DBL" ("Énum")
                w373 = "OCV" ("section")
                n113 = call <userlib>:"Read_Param.vi"("Énum"=w371, "errin"=w370, "section"=w373, "key"="ZEN79min30") -> ("error out"=w374:errorcluster, "dbl"=w369:dbl)  [unwired: 3 in, 3 out]
                n114 = call <userlib>:"Read_Param.vi"("Énum"=w371, "errin"=w374, "section"=w373, "key"="ZEN79max30") -> ("error out"=w367:errorcluster, "dbl"=w368:dbl)  [unwired: 3 in, 3 out]
              }
            }
          }
          frame "ZEN82" {
            n115 = case shown="True" w376 {
              tunnel: w380 -> [w384 w394]
              tunnel: [w383 w393] -> w379
              tunnel: [w382 w392] -> w378
              tunnel: [w381 w391] -> w377
              frame False {
                w385 = enum16{"STR", "DBL", "U32"}."DBL" ("Énum")
                w387 = "OCV" ("section")
                n116 = call <userlib>:"Read_Param.vi"("Énum"=w385, "errin"=w384, "section"=w387, "key"="ZEN82min70") -> ("error out"=w388:errorcluster, "dbl"=w381:dbl)  [unwired: 3 in, 3 out]
                n117 = call <userlib>:"Read_Param.vi"("Énum"=w385, "errin"=w388, "section"=w387, "key"="ZEN82max70") -> ("error out"=w383:errorcluster, "dbl"=w382:dbl)  [unwired: 3 in, 3 out]
              }
              frame True {
                w395 = enum16{"STR", "DBL", "U32"}."DBL" ("Énum")
                w397 = "OCV" ("section")
                n118 = call <userlib>:"Read_Param.vi"("Énum"=w395, "errin"=w394, "section"=w397, "key"="ZEN82min30") -> ("error out"=w398:errorcluster, "dbl"=w391:dbl)  [unwired: 3 in, 3 out]
                n119 = call <userlib>:"Read_Param.vi"("Énum"=w395, "errin"=w398, "section"=w397, "key"="ZEN82max30") -> ("error out"=w393:errorcluster, "dbl"=w392:dbl)  [unwired: 3 in, 3 out]
              }
            }
          }
          frame "ZEN84" {
            n120 = case shown="True" w399 {
              tunnel: w403 -> [w407 w416]
              tunnel: [w406 w415] -> w402
              tunnel: [w405 w414] -> w401
              tunnel: [w404 w413] -> w400
              frame False {
                w408 = enum16{"STR", "DBL", "U32"}."DBL" ("Énum")
                w410 = "OCV" ("section")
                n121 = call <userlib>:"Read_Param.vi"("Énum"=w408, "errin"=w407, "section"=w410, "key"="ZEN84min70") -> ("error out"=w411:errorcluster, "dbl"=w404:dbl)  [unwired: 3 in, 3 out]
                n122 = call <userlib>:"Read_Param.vi"("Énum"=w408, "errin"=w411, "section"=w410, "key"="ZEN84max70") -> ("error out"=w406:errorcluster, "dbl"=w405:dbl)  [unwired: 3 in, 3 out]
              }
              frame True {
                w417 = enum16{"STR", "DBL", "U32"}."DBL" ("Énum")
                w419 = "OCV" ("section")
                n123 = call <userlib>:"Read_Param.vi"("Énum"=w417, "errin"=w416, "section"=w419, "key"="ZEN84min30") -> ("error out"=w420:errorcluster, "dbl"=w413:dbl)  [unwired: 3 in, 3 out]
                n124 = call <userlib>:"Read_Param.vi"("Énum"=w417, "errin"=w420, "section"=w419, "key"="ZEN84max30") -> ("error out"=w415:errorcluster, "dbl"=w414:dbl)  [unwired: 3 in, 3 out]
              }
            }
          }
        }
        n125 = flat-sequence {
          tunnel: [w278] -> w257
          tunnel: w258 -> [w278]
          frame #0 {
            n126 = call <userlib>:"FGV_Image.vi"("Énum"=FGV."SET", "IN"="OCV") -> ()  [unwired: 9 in, 1 out]
          }
        }
        n127 = global write "OP400ZP_OCVmax.vi" "OCVmax"(w261) -> ()
        n128 = global write "OP400ZP_OCVmin.vi" "OCVmin"(w262) -> ()
        n129 = while {
          tunnel: [w301] -> w256
          shift-right: [w303] -> w273
          shift-left: w257 -> [w302]
          tunnel: w262 -> [w286]
          tunnel: w261 -> [w284]
          tunnel: [w283] -> w263
          stop <- w283 stop-if-true
          n130 = global read "VG_MX5060.vi" "MX5060"() -> (w300:string)
          n131 = call-poly "VISA Configure Serial Port"("VISA resource name"=w300, "baud rate (9600)"=u32 4800, "error in (no error)"=w302) -> ("VISA resource name out"=w297:refnum<visa-resource-name>, "error out"=w298:errorcluster)  [unwired: 11 in]
          n132 = Concatenate Strings(":READ?" ("chaîne"), "\r\n") -> (w289:string)
          n133 = VISA Write(VISA resource name=w297, write buffer=w289, error in (no error)=w298) -> (VISA resource name out=w295:refnum<visa-resource-name>, error out=w296:errorcluster)  [unwired: 1 out]
          n134 = VISA Read(VISA resource name=w295, byte count=u32 30 ("nombre d'octets"), error in (no error)=w296) -> (VISA resource name out=w293:refnum<visa-resource-name>, read buffer=w287:string, error out=w294:errorcluster)  [unwired: 1 out]
          n135 = Match Pattern(string=w287, regular expression=" VACDC " ("expression régulière")) -> (before substring=w301:string)  [unwired: 1 in, 3 out]
          n136 = Fract/Exp String To Number(string=w301) -> (number=w285:dbl)  [unwired: 3 in, 1 out]
          n137 = call <vilib>:"Clear Errors.vi"("error in (no error)"=w294, "specific error code to clear (0: all)"=-1073807339) -> ("error out"=w282:errorcluster)  [unwired: 4 in, 1 out]
          n138 = In Range and Coerce(upper limit=w284, x=w285, lower limit=w286) -> (In Range?=w283:bool)  [unwired: 1 out]
          n139 = VISA Close(VISA resource name=w293, error in (no error)=w282) -> (error out=w303:errorcluster)
        }
        n140 = local read "BDD"() -> (w267:T3)
        n141 = Concatenate Strings("Vpack;" ("chaîne"), w256) -> (w271:string)
        n142 = Bundle By Name(cluster=w267, "OCV"=w256) -> (w266:T3)
        n143 = call "Log_basic.vi"("errin"=w277, "chaîne"=w271, "in"=w276) -> ("sortie d'erreur"=w274:errorcluster, "refnum en sortie"=w275:refnum<file>)  [unwired: 7 in]
        n144 = local write "BDD"(w266) -> ()
        n145 = Select ("Sélectionner")(t=w264, s=w263, f=OP400ZP_state."Crash" ("cas faux")) -> (s? t:f=w269:T5)
      }
      frame "DataDyn" {
        w459 = OP400ZP_state."Demontage"  # Énum
        # "Divers data du pack"
        n146 = global read "ZENTYPE.vi" "ZENTYPE"() -> (w422:string)
        n147 = local write "TOP"("Analyse des CMU ..." ("TOP")) -> ()
        n148 = call <userlib>:"Read_Param.vi"("Énum"=enum16{"STR", "DBL", "U32"}."DBL", "errin"=w433, "section"="NbModule", "key"=w422) -> ("error out"=w432:errorcluster, "dbl"=w429:dbl)  [unwired: 3 in, 3 out]
        n149 = To Byte Integer(number=w429) -> (8bit integer=w428:i8)
        n150 = call "OUINON.vi"("errin"=w432, "image"="ISOPDU") -> ("error out"=w435:errorcluster, "OUI/NON"=w434:bool)  [unwired: 8 in]
        n151 = case shown="True" w434 {
          tunnel: w435 -> [w484 w502]
          tunnel: [w483 w508] -> w430
          tunnel: [w482 w507] -> w424
          tunnel: [w481 w506] -> w425
          tunnel: [w480 w509] -> w427
          tunnel: [w479 w510] -> w426
          tunnel: [w478 w505] -> _
          tunnel: [FALSE ("MCU") w505] -> _
          tunnel: w428 -> [w469 _]
          tunnel: w428 -> [_ w497]
          frame False {
            # "A supprimer avec nouvelle config ISO SPI"
            n152 = call <userlib>:"FGV_Image.vi"("Énum"=FGV."SET", "IN"="J1ON") -> ("OUT"=w472:string)  [unwired: 9 in]
            n153 = call "OUINON.vi"("errin"=w484, "image"=w472) -> ("error out"=w471:errorcluster)  [unwired: 8 in, 1 out]
            n154 = property on="progression" class="Slide (strict)"(error in=w471, "Visible"=TRUE, "Value"=u8 0 ("progression")) -> (error out=w476:errorcluster)  [unwired: 1 in, 1 out]
            n155 = flat-sequence {
              tunnel: [w494] -> w483
              tunnel: [w493] -> w482
              tunnel: [w492] -> w481
              tunnel: [w491] -> w480
              tunnel: [w490] -> w479
              tunnel: [w489] -> w478
              tunnel: w476 -> [w488]
              tunnel: w469 -> [_]
              frame #0 {
                n156 = call <userlib>:"SCAN CMU.vi"("errin"=w488, "Nb modules"=i16 26) -> ("errout"=w494:errorcluster, "# température + #tension OK?"=w489:bool, "Vmin"=w493:dbl, "Vmax"=w492:dbl, "Tmin"=w490:dbl, "Tmax"=w491:dbl)  [unwired: 4 out]
                n157 = call <userlib>:"FGV_Image.vi"("Énum"=FGV."SET", "IN"="DataDyn") -> ()  [unwired: 9 in, 1 out]
              }
            }
          }
          frame True {
            w505 = TRUE ("MCU")
            # "Ne répond pas à IDN.."
            n158 = global read "VG_ARDUINO.vi" "ARDUINO"() -> (w495:string)
            n159 = while {
              tunnel: [w524] -> _
              shift-right: [w525] -> w499
              shift-left: w502 -> [w527]
              tunnel: w495 -> [w518]
              i -> [w521]
              stop <- w526 stop-if-true
              n160 = call "detectISOSPI.vi"("errin"=w527, "VISA resource name"=w518) -> ("sortie d'erreur"=w525:errorcluster, "cas faux"=w524:string)  [unwired: 8 in]
              n161 = Greater? ("Supérieur ?")(x=w521, y=2) -> (0:w519:bool)
              n162 = Not Equal? ("Différents ?")(x="", y=w524) -> (x != y?=w522:bool)
              n163 = Compound Arithmetic op=OR ("Opérateur arithmétique")(w522, w519, w525) -> (w526:bool)
            }
            n164 = while {
              shift-right: [w515] -> _
              shift-left: 0.0 -> [w517]
              stop <- w516 stop-if-true
              n165 = Wait (ms)(milliseconds to wait=u32 7) -> ()  [unwired: 1 out]
              n166 = Increment(x=w517) -> (x+1=w515:dbl)
              n167 = global write "VG_progressBar.vi" "progression"(w515) -> ()
              n168 = Equal?(x=w515, y=1000) -> (x = y?=w516:bool)
            }
            n169 = property on="progression" class="Slide (strict)"(error in=w499, "Visible"=TRUE, "Value"=u8 0 ("progression")) -> (error out=w498:errorcluster)  [unwired: 1 in, 1 out]
            n170 = call <userlib>:"BriqueISOSPI_OP400.vi"("errin"=w498, "nbmodule"=w497, "visain"=w495) -> ("errout"=w508:errorcluster, "TCellmax"=w509:dbl, "VCellmax"=w511:dbl, "TCellmin"=w510:dbl, "VCellmin"=w512:dbl)  [unwired: 2 in, 2 out]
            n171 = expression code="x*1000"(w512) -> (w507:dbl)
            n172 = expression code="x*1000"(w511) -> (w506:dbl)
            n173 = call <userlib>:"FGV_Image.vi"("Énum"=FGV."SET", "IN"="DataDyn") -> ()  [unwired: 9 in, 1 out]
          }
        }
        n174 = global read "IS30%.vi" "VG IS30% ?"() -> (w444:bool)
        n175 = call "OP400ZP_Test_DataDyn.vi"("Tcell Min (°C)"=w426, "is30%?"=w444, "MCU"=TRUE, "Tcell Max (°C)"=w427, "Température usine (°C)"=21.0, "errin"=w430, "testname"="Dyn;", "Vcell Min (V)"=w424, "Vcell Max (V)"=w425) -> ("pass"=w438:bool, "datalog"=w464:string, "Cluster"=w449:T9, "errout"=w440:errorcluster)  [unwired: 2 in, 1 out]
        n176 = call "Log_basic.vi"("errin"=w467, "date?"=TRUE, "chaîne"=w464, "in"=w468) -> ("sortie d'erreur"=w466:errorcluster, "refnum en sortie"=w465:refnum<file>)  [unwired: 6 in]
        n177 = Unbundle By Name(w449) -> ("1_TCellmin"=w448:string, "1_TCellmax"=w447:string, "1_VCellmin"=w446:string, "1_VCellmax"=w445:string, "1_TUsine"=w443:string, "1_DeltaV"=w442:string, "1_DeltaT"=w441:string)
        n178 = property on="progression" class="Slide (strict)"(error in=w440, "Visible"=FALSE, "Value"=u8 0 ("progression")) -> (error out=w439:errorcluster)  [unwired: 1 in, 1 out]
        n179 = local read "BDD"() -> (w450:T3)
        n180 = Bundle By Name(cluster=w450, "Tmin"=w448, "Tmax"=w447, "Vmin"=w446, "Vmax"=w445, "Tusine"=w443, "DeltaV"=w442, "DeltaT"=w441) -> (w451:T3)
        n181 = local write "BDD"(w451) -> ()
        n182 = call "OP400ZP_refaire.vi"("refaire"=w461, "Pédale"=FALSE, "Cas OK"=w459, "errin"=w439, "test ok ?"=w438) -> ("errout"=w437:errorcluster, "OUT"=w460:T5)  [unwired: 5 in]
      }
      frame "Montage" {
        w529 = OP400ZP_state."Conti"  # Énum
        # "montage du produit sur le banc"
        n183 = call "OUINON.vi"("errin"=w537, "image"="Montage" ("IN")) -> ("error out"=w536:errorcluster, "OUI/NON"=w531:bool)  [unwired: 8 in]
        n184 = Select ("Sélectionner")(t=w529, s=w531, f=OP400ZP_state."Crash" ("cas faux")) -> (s? t:f=w530:T5)
        n185 = local write "TOP"("Montage du pack" ("TOP")) -> ()
      }
      frame "Demontage" {
        w553 = OP400ZP_state."Next"  # Énum
        n186 = call "OUINON.vi"("errin"=w556, "image"="Demontage" ("IN")) -> ("error out"=w550:errorcluster, "OUI/NON"=w544:bool)  [unwired: 8 in]
        n187 = Select ("Sélectionner")(t=w553, s=w544, f=OP400ZP_state."Crash" ("cas faux")) -> (s? t:f=w552:T5)
        n188 = Refnum to Path(1:w541) -> (0:w540:path)
        n189 = call <userlib>:"TEMPS_TEST.vi"("errin"=w543, "pathin"=w540) -> ("error out"=w542:errorcluster, "Delay calculé"=w539:string)  [unwired: 8 in]
        n190 = flat-sequence {
          tunnel: [FALSE] -> w558
          tunnel: w550 -> [_]
          frame #0 {
          }
        }
        n191 = Select ("Sélectionner")(t="1", s=w544, f="0" ("cas faux")) -> (s? t:f=w546:string)
        n192 = local write "TOP"("Demontez le pack" ("TOP")) -> ()
        n193 = local read "BDD"() -> (w549:T3)
        n194 = Bundle By Name(cluster=w549, "Pass"=w546, "TempsTest"=w539) -> (w545:T3)
        n195 = local write "BDD"(w545) -> ()
      }
      frame "Crash" {
        # "\\\\forseepower.com\\fr\\040 Production\\FR7 - Poitiers\\06 Production\\05. Electronique\\Documents Control lib\\Archives\\ZEN PLUS"
        n196 = Close File(refnum=w561, error in=w577) -> (path=w563:path, error out=w582:errorcluster)
        n197 = Refnum to Path(1:w561) -> (0:w560:path)
        n198 = call <userlib>:"waitXms.vi"("attente (ms)"=u32 500, "errin"=w582) -> ("errout"=w576:errorcluster)  [unwired: 13 in]
        n199 = local read "PN"() -> (w569:string)
        n200 = local read "SN"() -> (w574:string)
        n201 = call <userlib>:"FGV_Image.vi"("Énum"=FGV."SET", "IN"="TeamLeader") -> ()  [unwired: 9 in, 1 out]
        n202 = call <userlib>:"TEMPS_TEST.vi"("errin"=w576, "pathin"=w560) -> ("error out"=w564:errorcluster, "Delay calculé"=w562:string)  [unwired: 8 in]
        n203 = Concatenate Strings(w569, "-SN" ("chaîne"), w574) -> (w572:string)
        n204 = call "OP400ZP_NouveauDossier.vi"("entrée d'erreur (pas d'erreur)"=w564, "Nom du repertoire (PN SN)"=w572, "Network before adding a new folder"=path "\\\\forseepower.com\\fr/040 Production/FR7 - Poitiers/06 Production/05. Electronique/Documents Control lib/Archives/ZEN PLUS" ("chemin de la cible (utiliser une boîte de dialogue)")) -> ("sortie d'erreur"=w575:errorcluster, "Network after adding a new folder"=w570:path)  [unwired: 7 in]
        n205 = Copy ("Copier")(8:w575, 10:w570, 11:w563) -> (0:w580:errorcluster)  [unwired: 2 in, 2 out]
        n206 = call "PvgeneratorOP400.vi"("errin"=w580, "network"=w570, "path in"=w563) -> ("sortie d'erreur"=w579:errorcluster, "network out"=w578:path)  [unwired: 3 in, 4 out]
        n207 = call "POP_GOOGLE.vi"("error in"=w579, "chemin"=w578) -> ("error out"=w565:errorcluster)  [unwired: 8 in, 1 out]
        n208 = local write "TOP"("Crash..." ("TOP")) -> ()
        n209 = local read "BDD"() -> (w567:T3)
        n210 = Bundle By Name(cluster=w567, "Pass"="0" ("Résultat final"), "TempsTest"=w562) -> (w568:T3)
        n211 = local write "BDD"(w568) -> ()
      }
      frame "Next" {
        n212 = Close File(refnum=w611, error in=w610) -> (path=w592:path, error out=w607:errorcluster)
        n213 = call <userlib>:"waitXms.vi"("attente (ms)"=u32 500, "errin"=w607) -> ("errout"=w589:errorcluster)  [unwired: 13 in]
        n214 = local read "PN"() -> (w601:string)
        n215 = local read "SN"() -> (w600:string)
        n216 = Concatenate Strings(w601, "-SN" ("chaîne"), w600) -> (w598:string)
        n217 = call "OP400ZP_NouveauDossier.vi"("entrée d'erreur (pas d'erreur)"=w589, "Nom du repertoire (PN SN)"=w598, "Network before adding a new folder"=path "\\\\forseepower.com\\fr/040 Production/FR7 - Poitiers/06 Production/05. Electronique/Documents Control lib/Archives/ZEN PLUS" ("chemin de la cible (utiliser une boîte de dialogue)")) -> ("sortie d'erreur"=w602:errorcluster, "Network after adding a new folder"=w597:path)  [unwired: 7 in]
        n218 = Copy ("Copier")(8:w602, 10:w597, 11:w592) -> (0:w605:errorcluster)  [unwired: 2 in, 2 out]
        n219 = local read "BDD"() -> (w593:T3)
        n220 = call "PvgeneratorOP400.vi"("errin"=w605, "BDD 3"=w593, "network"=w597, "path in"=w592) -> ("sortie d'erreur"=w604:errorcluster, "network out"=w603:path, "chaîne concaténée"=→"INSERT INTO":string, "error out"=→"error out":errorcluster)  [unwired: 2 in, 2 out]
        n221 = call "OUINON.vi"("errin"=w614, "image"="Next" ("IN")) -> ("error out"=w613:errorcluster, "OUI/NON"=w594:bool)  [unwired: 8 in]
        n222 = call "POP_GOOGLE.vi"("error in"=w604, "chemin"=w603) -> ("error out"=w595:errorcluster)  [unwired: 8 in, 1 out]
        n223 = Select(t=OP400ZP_state."Scan" ("Énum"), s=w594, f=OP400ZP_state."Null" ("Énum")) -> (s? t:f=w612:T5)
      }
      frame "Sealing" {
        n224 = disable-structure shown="Désactivé" {
          disable-tunnel: w623 -> [w647 _]
          disable-tunnel: [w646 _] -> w622
          disable-tunnel: w621 -> [w645 _]
          disable-tunnel: [w644 _] -> w620
          disable-tunnel: [w638 _] -> w619
          disable-tunnel: [w637 _] -> w618
          disable-tunnel: w616 -> [w634 _]
          frame Disabled {
            w636 = OP400ZP_state."Montage" ("Cas OK")
            n225 = call "Test étancheité"("Enable"=TRUE, "error in (no error)"=w634) -> ("Etancheité  (Pa)"=w628:dbl, "error out"=w641:errorcluster)  [unwired: 15 in, 1 out]
            n226 = call <userlib>:"FGV_Image.vi"("Énum"=FGV."SET", "IN"="Sealing") -> ()  [unwired: 9 in, 1 out]
            n227 = call <vilib>:"Application Directory.vi"() -> ("Application Directory"=w643:path)
            n228 = call <userlib>:"Read_Param.vi"("Énum"=enum16{"STR", "DBL", "U32"}."DBL", "errin"=w641, 9:w643, "section"="Sealing", "key"="Max") -> ("error out"=w639:errorcluster, "dbl"=w627:dbl)  [unwired: 2 in, 3 out]
            n229 = In Range and Coerce ("Dans la gamme")(upper limit=w627, x=w628, lower limit=0.0 ("limite inférieure")) -> (In Range?=w625:bool)  [unwired: 1 out]
            n230 = call "OP400ZP_refaire.vi"("refaire"=OP400ZP_state."Sealing", "Cas OK"=w636, "errin"=w639, "test ok ?"=w625) -> ("errout"=w638:errorcluster, "OUT"=w637:T5)  [unwired: 6 in]
            n231 = Equal?(x=w637, y=w636) -> (x = y?=w635:bool)
            n232 = case shown="True" w635 {
              tunnel: w647 -> [w649 w657]
              tunnel: [w649 w656] -> w646
              tunnel: w645 -> [w648 w655]
              tunnel: [w648 w654] -> w644
              tunnel: w628 -> [_ w653]
              frame False {
              }
              frame True {
                n233 = Number To Decimal String(number=w653) -> (decimal integer string=w650:string)  [unwired: 1 in]
                n234 = local read "BDD"() -> (w652:T3)
                n235 = Bundle By Name(cluster=w652, "Sealing"=w650) -> (w651:T3)
                n236 = Concatenate Strings("Sealing;" ("chaîne"), w650) -> (w659:string)
                n237 = call "Log_basic.vi"("errin"=w657, "date?"=TRUE, "chaîne"=w659, "in"=w655) -> ("sortie d'erreur"=w656:errorcluster, "refnum en sortie"=w654:refnum<file>)  [unwired: 6 in]
                n238 = local write "BDD"(w651) -> ()
              }
            }
            n239 = local write "TOP"("Saisir la valeur du sealing pack" ("TOP")) -> ()
          }
          frame Enabled {
          }
        }
      }
      frame "Comext" {
        n240 = call "OUINON.vi"("errin"=w665, "image"="Comext" ("IN")) -> ("error out"=w664:errorcluster, "OUI/NON"=w661:bool)  [unwired: 8 in]
        n241 = case shown="True" w661 {
          tunnel: w674 -> [w679 w691]
          tunnel: w673 -> [w678 w690]
          tunnel: [w678 w689] -> w672
          tunnel: [w679 w688] -> w671
          tunnel: [OP400ZP_state."Crash" ("OUT") w687] -> w670
          tunnel: w669 -> [_ w686]
          tunnel: [w676 w685] -> w668
          tunnel: w667 -> [_ _]
          tunnel: w664 -> [w676 w683]
          tunnel: [w677 w682] -> w663
          tunnel: w662 -> [w677 w682]
          frame False {
          }
          frame True {
            w704 = OP400ZP_state."Demontage"  # Énum
            (unwired) "Refaire" ("image")
            n242 = local read "PN"() -> (w702:string)
            n243 = call <vilib>:"Application Directory.vi"() -> ()  [unwired: 1 out]
            n244 = call <userlib>:"Read_Param.vi"("Énum"=enum16{"STR", "DBL", "U32"}."U32", "errin"=w683, "section"="DataDyn", "key"=w702) -> ("error out"=w697:errorcluster, "U32"=w700:u32)  [unwired: 3 in, 3 out]
            n245 = property on="progression" class="Slide (strict)"(error in=w697, "Visible"=TRUE, "Value"=u8 0 ("progression")) -> (error out=w696:errorcluster)  [unwired: 1 in, 1 out]
            n246 = call <userlib>:"FGV_Image.vi"("Énum"=FGV."SET", "IN"="DataDyn") -> ()  [unwired: 9 in, 1 out]
            n247 = call <userlib>:"SCAN CMU.vi"("errin"=w696, "Nb modules"=w700) -> ("errout"=w713:errorcluster, "# température + #tension OK?"=w708:bool, "Vmin"=w712:dbl, "Vmax"=w711:dbl, "Tmin"=w709:dbl, "Tmax"=w710:dbl)  [unwired: 4 out]
            n248 = call "OP400ZP_Test_DataDyn.vi"("Tcell Min (°C)"=w709, "MCU"=w708, "Tcell Max (°C)"=w710, "Température usine (°C)"=21.0, "errin"=w713, "testname"="Comext;", "Vcell Min (V)"=w712, "Vcell Max (V)"=w711) -> ("pass"=w706:bool, "datalog"=w715:string, "errout"=w707:errorcluster)  [unwired: 3 in, 2 out]
            n249 = call "Log_basic.vi"("errin"=w691, "date?"=TRUE, "chaîne"=w715, "in"=w690) -> ("sortie d'erreur"=w688:errorcluster, "refnum en sortie"=w689:refnum<file>)  [unwired: 6 in]
            n250 = call "OP400ZP_refaire.vi"("refaire"=w686, "Pédale"=FALSE, "Cas OK"=w704, "errin"=w707, "test ok ?"=w706) -> ("errout"=w692:errorcluster, "OUT"=w687:T5)  [unwired: 5 in]
            n251 = property on="progression" class="Slide (strict)"(error in=w692, "Visible"=FALSE, "Value"=u8 0 ("progression")) -> (error out=w685:errorcluster)  [unwired: 1 in, 1 out]
          }
        }
      }
    }
    n252 = Wait (ms)(milliseconds to wait=u32 200 ("attente (ms)")) -> ()  [unwired: 1 out]
    n253 = case shown="False" w29 {
      selector: w29 -> [_ w36]
      frame False {
      }
      frame True {
        n254 = local write "STOP"(w36) -> ()
      }
    }
  }
  n255 = while {
    shift-right: [w724] -> _
    shift-left: errorcluster {"status"=FALSE, "code"=0, "source"=""} ("error out") -> [w723]
    tunnel: w7 -> [_]
    i -> [w717]
    stop <- w716 stop-if-true
    # "ici tu met l'image à jour si besoin"
    n256 = Wait (ms)(milliseconds to wait=u32 10 ("attente (ms)")) -> ()  [unwired: 1 out]
    n257 = call <userlib>:"FGV_Image.vi"("Énum"=FGV."GET") -> ("OUT"=w719:string)  [unwired: 10 in]
    n258 = Not Equal?(x=w719, y="") -> (x != y?=w720:bool)
    n259 = case shown="True" w720 {
      tunnel: [w726 w732] -> w724
      tunnel: w723 -> [w726 w731]
      tunnel: w719 -> [_ w730]
      frame False {
      }
      frame True {
        n260 = call <vilib>:"Application Directory.vi"() -> ("Application Directory"=w734:path)
        n261 = Path To String(path=w734) -> (string=w735:string)
        n262 = Concatenate Strings(w735, "\\Image\\" ("chaîne"), w730, ".jpg" ("chaîne")) -> (w728:string)
        n263 = String To Path(string=w728) -> (path=w733:path)
        n264 = call <userlib>:"FGV_Image.vi"("Énum"=FGV."RAZ") -> ()  [unwired: 10 in, 1 out]
        n265 = call <vilib>:"Read JPEG File.vi"("error in (no error)"=w731, "path to JPEG file"=w733) -> ("error out"=w732:errorcluster, "image data"=w738:T10)  [unwired: 7 in, 1 out]
        n266 = call <vilib>:"Draw Flattened Pixmap.vi"("image data"=w738) -> ("new picture"=w729:picture)  [unwired: 8 in]
        n267 = local write "DRAW"(w729) -> ()
      }
    }
    n268 = global read "VG_progressBar.vi" "progression"() -> (→"progression":dbl)
    n269 = local read "STOP"() -> (w716:bool)
    "Numérique" <- w717
  }
  n270 = while {
    shift-right: [w743] -> _
    shift-left: errorcluster {"status"=FALSE, "code"=0, "source"=""} ("error out") -> [w743]
    tunnel: [w739] -> w4
    stop <- w739 stop-if-true
    n271 = call "ARRET.vi"("arrêt"="arrêt") -> ("T button?"=w741:bool)  [unwired: 10 in]
    n272 = local read "STOP"() -> (w740:bool)
    n273 = Or(x=w740, y=w741) -> (x .or. y?=w739:bool)
  }
  n274 = Stop(stop? (T)=w4) -> ()
  n275 = Merge Errors(w20, w19) -> (→"errout":errorcluster)
  "STOP" <- w7
